vi "Log Results.vi"(0 "Log File Ref. In":refnum<file>, 2 "Results Name":string, 7 "Data Input":string[][](array[string]), 11 "error in":errorcluster) -> (4 "Log File Ref. Out":refnum<file>, 6 "Cancelled":bool, 15 "error out":errorcluster)   [LabVIEW 2024, in "dataLogger.lvlib"]
doc: "<B>Log Cussom Data</B> API. \n\nGets any 2D string array and log it in the created log file in CSV formatting"
uses:
  dataLogger.lvlib
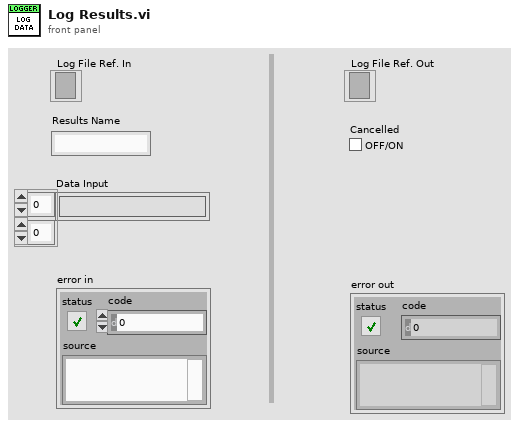
[diagram p1: front panel]
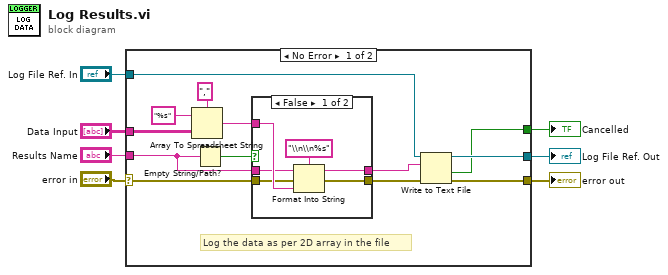
[diagram p0: block diagram]
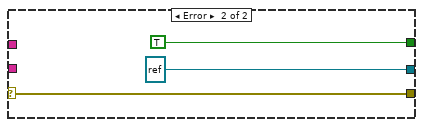
[diagram p3: hidden frame]
diagram:
  n1 = case shown="No Error" "error in" {
    selector: "error in" -> [w17 w31]
    tunnel: [w12 w31] -> w6
    tunnel: "Data Input" -> [w16 _]
    tunnel: [w10 TRUE ("cancelled")] -> w4
    tunnel: "Results Name" -> [w15 _]
    tunnel: [w11 refnum<file> refnum ("refnum out")] -> w2
    tunnel: "Log File Ref. In" -> [w8 _]
    frame No Error {
      # "Log the data as per 2D array in the file"
      n2 = Array To Spreadsheet String(delimiter (Tab)=",", array=w16, 3:"%s" ("format string")) -> (spreadsheet string=w18:string)
      n3 = Empty String/Path?(string/path=w15) -> (empty?=w14:bool)
      n4 = case shown="False" w14 {
        tunnel: [w26 w27] -> w13
        tunnel: w18 -> [w24 w28]
        tunnel: [w23 w28] -> w9
        tunnel: w17 -> [w22 w27]
        tunnel: w15 -> [w21 _]
        frame False {
          n5 = Format Into String(format string="\\n\\n%s", initial string=w21, error in=w22, w24) -> (resulting string=w23:string, error out=w26:errorcluster)
        }
        frame True {
        }
      }
      n6 = Write to Text File(file (use dialog)=w8, text=w9, error in=w13) -> (refnum out=w11:refnum<file>, cancelled=w10:bool, error out=w12:errorcluster)  [unwired: 1 in]
    }
    frame Error {
    }
  }
  "error out" <- w6
  "Cancelled" <- w4
  "Log File Ref. Out" <- w2
